vi "BurstTrain-Create (Continuous).vi"(0 "State In":T1, 5 "Burst Rate (Hz)":dbl=1.0 min=1.0 max=40.0, 9 "Fs (Hz)":dbl, 11 "Npts":i32) -> (4 "State Out":T1, 8 "Buffer":dbl[](array[numeric]), 15 "New period?":bool)   [LabVIEW 2015]
uses:
  Burst Train-Continuous State.ctl
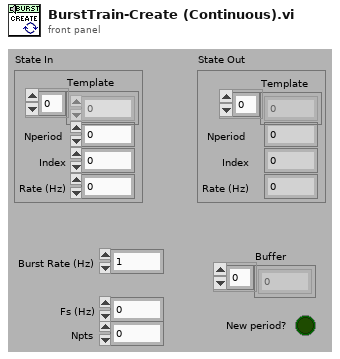
[diagram p1: front panel]
types:
  T1 = typedef "Burst Train-Continuous State.ctl" = cluster{"Template":dbl[], "Nperiod":i32, "Index":i32, "Rate (Hz)":dbl}
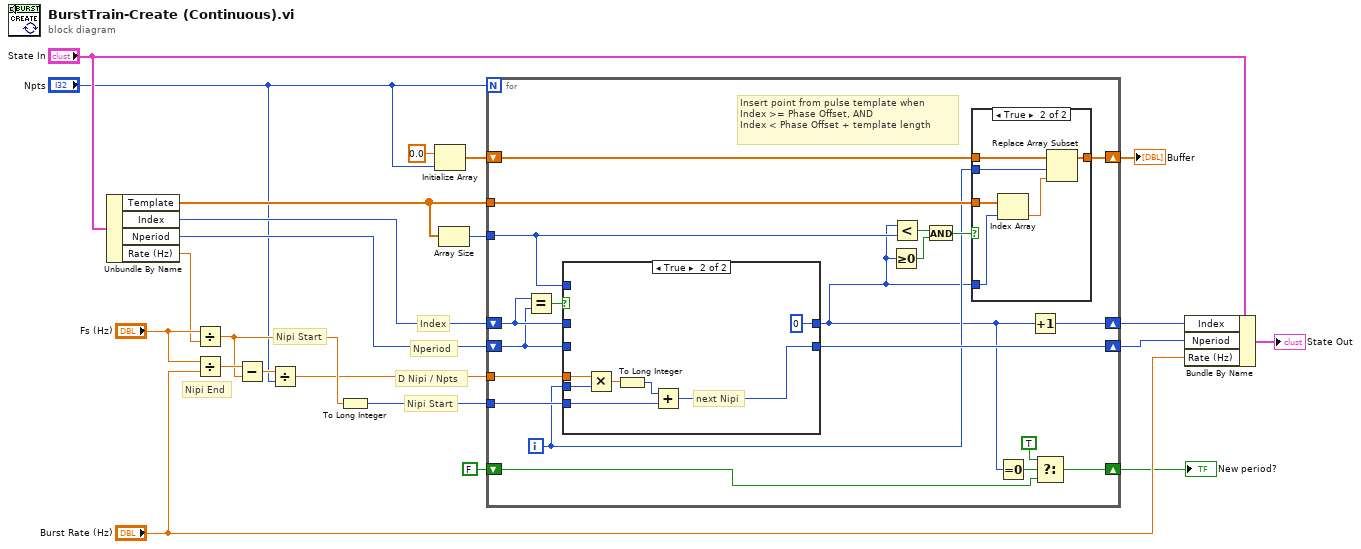
[diagram p0: block diagram]
diagram:
  # "Nperiod"
  # "Index"
  # "Nipi Start"
  # "D Nipi / Npts"
  # "Nipi End"
  # "Nipi Start"
  n1 = Unbundle By Name("State In") -> ("Template"=w8:dbl[], "Index"=w11:i32, "Nperiod"=w9:i32, "Rate (Hz)"=w17:dbl)
  n2 = Divide(x="Fs (Hz)", y=w17) -> (x/y=w14:dbl)
  n3 = Divide(x="Fs (Hz)", y="Burst Rate (Hz)") -> (x/y=w15:dbl)
  n4 = Subtract(x=w15, y=w14) -> (x-y=w13:dbl)
  n5 = Divide(x=w13, y="Npts") -> (x/y=w12:dbl)
  n6 = To Long Integer(number=w14) -> (32bit integer=w16:i32)
  n7 = Initialize Array(0.0 ("element"), "Npts") -> (w10:dbl[])
  n8 = Array Size(array=w8) -> (size(s)=w7:i32)
  n9 = for {
    N: "Npts" -> [_]
    tunnel: w8 -> [w32]
    shift-right: [w36] -> w5
    shift-left: w11 -> [w40]
    tunnel: w16 -> [w42]
    tunnel: w12 -> [w41]
    shift-right: [w38] -> w4
    shift-left: w9 -> [w37]
    tunnel: w7 -> [w28]
    shift-right: [w29] -> w6
    shift-left: w10 -> [w31]
    shift-right: [w26] -> w1
    shift-left: FALSE -> [w24]
    i -> [w30]
    # "Insert point from pulse template when \nIndex >= Phase Offset, AND\nIndex < Phase Offset + template length"
    n10 = Equal?(x=w40, y=w37) -> (x = y?=w39:bool)
    n11 = case shown="True" w39 {
      tunnel: w42 -> [_ w58]
      tunnel: w41 -> [_ w56]
      tunnel: [w50 w52] -> w38
      tunnel: w40 -> [w51 _]
      tunnel: [w51 0 ("Index")] -> w23
      tunnel: w37 -> [w50 _]
      tunnel: w30 -> [_ w53]
      tunnel: w28 -> [_ _]
      frame False {
      }
      frame True {
        # "next Nipi"
        n12 = Multiply(x=w56, y=w53) -> (x*y=w57:dbl)
        n13 = To Long Integer(number=w57) -> (32bit integer=w55:i32)
        n14 = Add(x=w55, y=w58) -> (x+y=w52:i32)
      }
    }
    n15 = Greater Or Equal To 0?(x=w23) -> (x >= 0?=w34:bool)
    n16 = Less?(x=w23, y=w28) -> (x < y?=w35:bool)
    n17 = And(x=w35, y=w34) -> (x .and. y?=w33:bool)
    n18 = case shown="True" w33 {
      tunnel: w23 -> [_ w48]
      tunnel: w32 -> [_ w49]
      tunnel: w31 -> [w43 w47]
      tunnel: w30 -> [_ w45]
      tunnel: [w43 w44] -> w29
      frame False {
      }
      frame True {
        n19 = Index Array(array=w49, index=w48) -> (element=w46:dbl)
        n20 = Replace Array Subset(array=w47, new element=w46, index=w45) -> (w44:dbl[])
      }
    }
    n21 = Equal To 0?(x=w23) -> (x = 0?=w27:bool)
    n22 = Increment(x=w23) -> (x+1=w36:i32)
    n23 = Select(t=TRUE, s=w27, f=w24) -> (s? t:f=w26:bool)
  }
  "Buffer" <- w6
  "New period?" <- w1
  n24 = Bundle By Name(cluster="State In", "Index"=w5, "Nperiod"=w4, "Rate (Hz)"="Burst Rate (Hz)") -> (→"State Out":T1)
